vi "Scanner.vi"(4 "ProcValue":dbl, 6 "CircQuality":dbl, 7 "Threshold Limits":cluster{"Lower value":sgl, "Upper value":sgl}={"Lower value"=0.0, "Upper value"=255.0} {"Upper value" format="%.2f"; "Lower value" format="%.2f"}, 9 "AutoRange":bool, 10 "Image Dst":T1, 11 "Image In":T1) -> (1 "HorCenter":u16, 2 "VerCenter":u32, 3 "Image Out":T1)   [LabVIEW 2015]
uses:
  <vilib>/vision/Image Controls.llb/IMAQ Image.ctl
  <vilib>/vision/NI_Vision_Development_Module.lvlib
panel:
  out "CtualThresh":cluster{"Lower value":sgl, "Upper value":sgl}
  in  "CircleQualityThrs":dbl=1.0
  in  "RangeGain":sgl=5e-05 format="%#.8f"
  out "Sum 2":u8[][](graph)
  out "Threshold Range Out":cluster{"Lower value":sgl, "Upper value":sgl}={"Lower value"=128.0, "Upper value"=255.0} {"Upper value" format="%.2f"; "Lower value" format="%.2f"}
  in  "error in":errorcluster
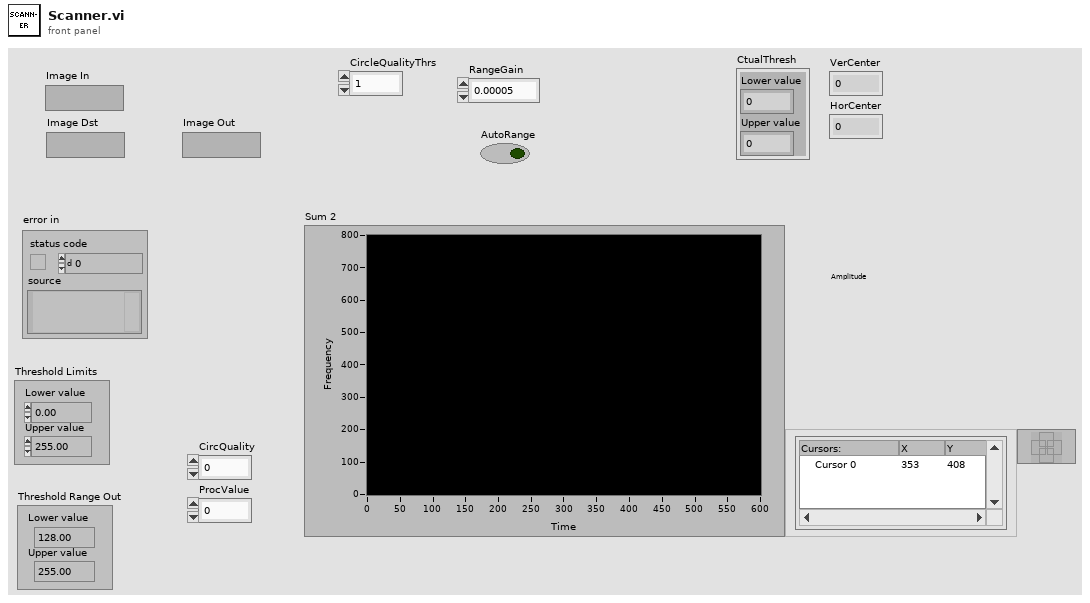
[diagram p1: front panel]
types:
  T1 = typedef "IMAQ Image.ctl" = refnum<image>
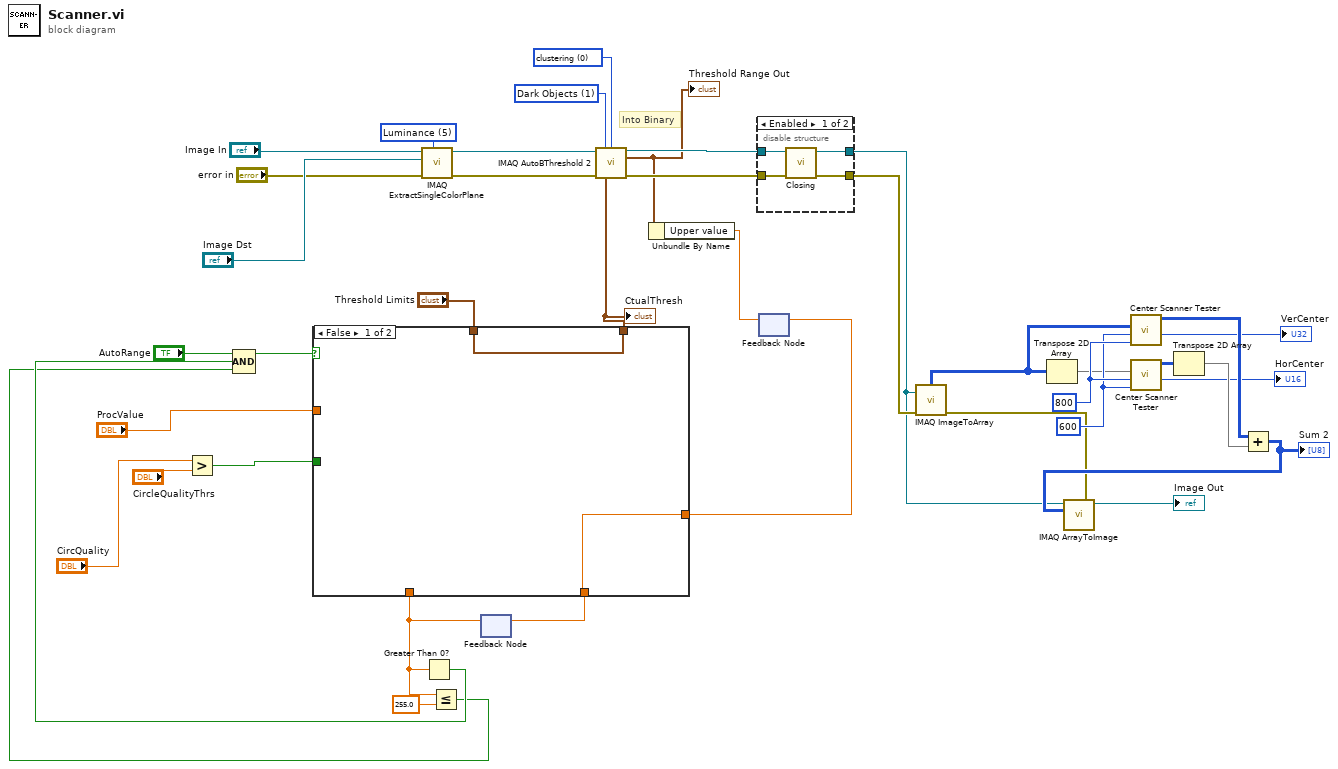
[diagram p0: block diagram]
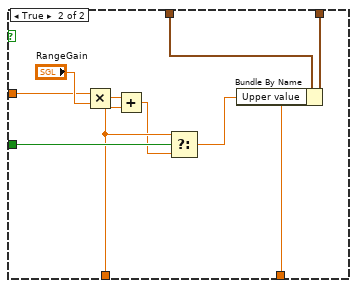
[diagram p3: hidden frame]
diagram:
  w36 = u16 800 ("Hight")
  w35 = u16 600 ("Width")
  w38 = u32 1 items=["Bright Objects", "Dark Objects"] ("Look For (Bright Objects)")
  w39 = 0 items=["clustering", "entropy", "metric", "moments", "inter-class variance"] ("Method")
  w40 = 5 items=["Red", "Green", "Blue", "Hue", "Saturation", "Luminance", "Value", "Intensity"] ("Color Plane")
  # "Into Binary"
  n1 = Greater?(x="CircQuality", y="CircleQualityThrs") -> (0:w13:bool)
  n2 = call "IMAQ ExtractSingleColorPlane"("Color Plane"=w40, "error in (no error)"="error in", "Image Dst"="Image Dst", "Image Src"="Image In") -> ("error out"=w24:errorcluster, "Image Dst Out"=w23:T1)  [unwired: 6 out]
  n3 = feedback #1() -> (w7:dbl)  [unwired: 1 in]
  n4 = Greater Than 0?(x=w7) -> (x > 0?=w8:bool)
  n5 = Less Or Equal?(x=w7, y=255.0) -> (x <= y?=w5:bool)
  n6 = Compound Arithmetic op=AND("AutoRange", w8, w5) -> (w9:bool)
  n7 = feedback #2() -> (w11:sgl)  [unwired: 1 in]
  n8 = case shown="False" w9 {
    tunnel: "Threshold Limits" -> [w42 w51]
    tunnel: [w42 w50] -> w15
    tunnel: [w41 w46] -> w18
    tunnel: w7 -> [_ w44]
    tunnel: w13 -> [_ w47]
    tunnel: "ProcValue" -> [_ w45]
    tunnel: w11 -> [w41 _]
    frame False {
    }
    frame True {
      n9 = Multiply(x=w45, y="RangeGain") -> (x*y=w48:dbl)
      n10 = Add(x=w48, y=w44) -> (x+y=w43:dbl)
      n11 = Select(t=w44, s=w47, f=w43) -> (s? t:f=w46:dbl)
      n12 = Bundle By Name(cluster=w51, "Upper value"=w46) -> (w50:cluster{"Lower value":sgl, "Upper value":sgl})
    }
  }
  "CtualThresh" <- w15
  n13 = feedback-in #1(w18) -> ()
  n14 = call "IMAQ AutoBThreshold 2"("Image Src"=w23, "Look For (Bright Objects)"=w38, "Method (clustering)"=w39, "error in (no error)"=w24, "Threshold Limits"=w15) -> ("Image Dst Out"=w31:T1, "Threshold Range Out"=w14:cluster{"Lower value":sgl, "Upper value":sgl}, "error out"=w30:errorcluster)  [unwired: 3 in, 5 out]
  "Threshold Range Out" <- w14
  n15 = Unbundle By Name(w14) -> ("Upper value"=w12:sgl)
  n16 = disable-structure shown="Enabled" {
    disable-tunnel: [w55 w56] -> w37
    disable-tunnel: w31 -> [w54 w57]
    disable-tunnel: w30 -> [w53 w56]
    disable-tunnel: [w52 w57] -> w20
    frame Enabled {
      n17 = call "Closing.vi"("error in (no error)"=w53, "Refnum in"=w54) -> ("error out"=w55:errorcluster, "Refnum out"=w52:T1)  [unwired: 8 in]
    }
    frame Disabled {
    }
  }
  n18 = feedback-in #2(w12) -> ()
  n19 = call "IMAQ ImageToArray"("error in (no error)"=w37, "Image"=w20) -> ("error out"=w19:errorcluster, "Image Pixels (U8)"=w34:u8[][])  [unwired: 2 in, 3 out]
  n20 = Transpose 2D Array(2D array=w34) -> (transposed array=w33:u8[][])
  n21 = call "Center Scanner Tester.vi"("Hight"=w36, "Width"=w35, "ImageIn"=w34) -> ("HorCenter"=→"VerCenter":u16, "ImgOut"=w29:u8[][])  [unwired: 7 in]
  n22 = call "Center Scanner Tester.vi"("Hight"=w35, "Width"=w36, "ImageIn"=w33) -> ("HorCenter"=→"HorCenter":u16, "ImgOut"=w28:u8[][])  [unwired: 7 in]
  n23 = Transpose 2D Array(2D array=w28) -> (transposed array=w27:u8[][])
  n24 = Add(x=w29, y=w27) -> (x+y=w22:u8[][])
  "Sum 2" <- w22
  n25 = call "IMAQ ArrayToImage"("error in (no error)"=w19, "Image Pixels (U8)"=w22, "Image"=w20) -> ("Image Out"=→"Image Out":T1)  [unwired: 7 in, 1 out]
